vi "Check Stage Limit.vi"(7 "Lane length (mm)":dbl, 8 "error in (no error)":errorcluster, 9 "Lanes":i32, 10 "Fields":i32, 11 "Application in":refnum<class "Application.lvclass">) -> (0 "error out":errorcluster, 2 "In Range?":bool, 3 "Application out":refnum<class "Application.lvclass">)   [LabVIEW 2023, in "Application.lvlib" / "Application.lvclass"]
uses:
  Application.lvclass
  Application.lvclass/Application.ctl
  Resources/GLOBAL/GLOBAL Experiment Metadata.vi
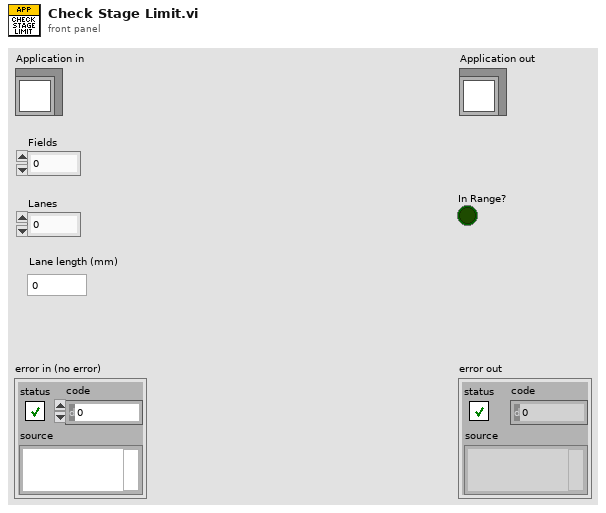
[diagram p1: front panel]
types:
  T1 = typedef "Stage Position.ctl" = cluster{"X (mm)":dbl, "Y (mm)":dbl, "Z (mm)":dbl}
  T2 = cluster{"Y Min":dbl, "Y Max":dbl, "X Min":dbl, "X Max":dbl}
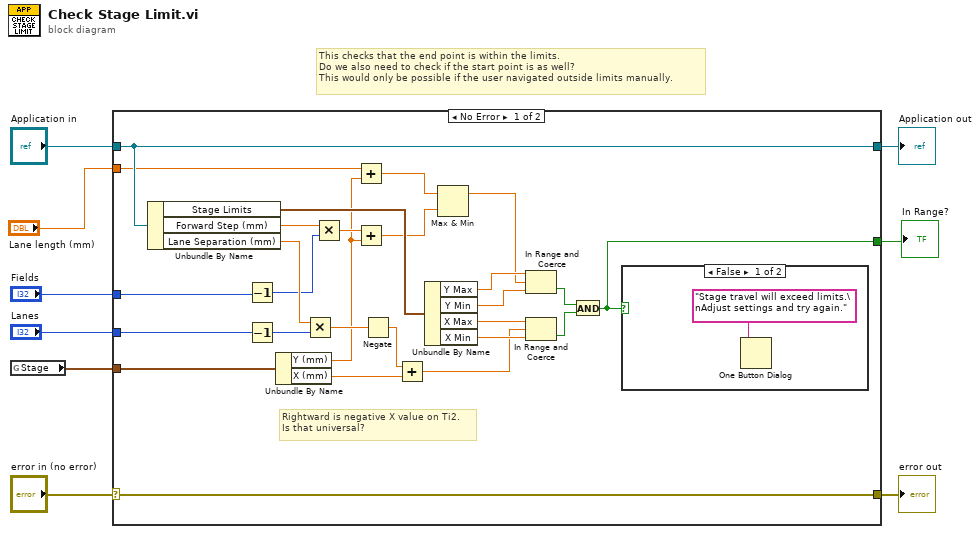
[diagram p0: block diagram]
diagram:
  # "This checks that the end point is within the limits.\nDo we also need to check if the start point is as well?\nThis would only be possible if the user navigated outside limits manually."
  n1 = global read "GLOBAL Experiment Metadata.vi" "Stage"() -> (w2:T1)
  n2 = case shown="No Error" "error in (no error)" {
    selector: "error in (no error)" -> [w36 w39]
    tunnel: [w36 w39] -> w8
    tunnel: [w35 w38] -> w6
    tunnel: "Application in" -> [w35 w38]
    tunnel: [w27 _] -> w5
    tunnel: "Fields" -> [w17 _]
    tunnel: "Lanes" -> [w16 _]
    tunnel: w2 -> [w10 _]
    tunnel: "Lane length (mm)" -> [w12 _]
    frame No Error {
      # "Rightward is negative X value on Ti2.\nIs that universal?"
      n3 = Unbundle By Name(w35) -> ("Stage Limits"=w32:T2, "Forward Step (mm)"=w26:dbl, "Lane Separation (mm)"=w22:dbl)
      n4 = Decrement(x=w17) -> (x-1=w18:i32)
      n5 = Decrement(x=w16) -> (x-1=w19:i32)
      n6 = Unbundle By Name(w10) -> ("Y (mm)"=w11:dbl, "X (mm)"=w23:dbl)
      n7 = Multiply(x=w22, y=w19) -> (x*y=w21:dbl)
      n8 = Multiply(x=w26, y=w18) -> (x*y=w25:dbl)
      n9 = Add(x=w12, y=w11) -> (x+y=w13:dbl)
      n10 = Add(x=w25, y=w11) -> (x+y=w14:dbl)
      n11 = Negate(x=w21) -> (-x=w20:dbl)
      n12 = Add(x=w20, y=w23) -> (x+y=w24:dbl)
      n13 = Unbundle By Name(w32) -> ("Y Max"=w31:dbl, "Y Min"=w30:dbl, "X Max"=w29:dbl, "X Min"=w28:dbl)
      n14 = Max & Min(x=w13, y=w14) -> (max(x,y)=w15:dbl)  [unwired: 1 out]
      n15 = In Range and Coerce(upper limit=w31, x=w15, lower limit=w30) -> (In Range?=w34:bool)  [unwired: 1 out]
      n16 = In Range and Coerce(upper limit=w29, x=w24, lower limit=w28) -> (In Range?=w33:bool)  [unwired: 1 out]
      n17 = And(x=w34, y=w33) -> (x .and. y?=w27:bool)
      n18 = case shown="False" w27 {
        frame False {
          n19 = One Button Dialog(message="Stage travel will exceed limits.\nAdjust settings and try again.") -> ()  [unwired: 1 in, 1 out]
        }
        frame True {
        }
      }
    }
    frame Error {
    }
  }
  "error out" <- w8
  "Application out" <- w6
  "In Range?" <- w5
